vi "Is Possible.vi"(8 "error in (no error)":errorcluster, 10 "Cubes":T1, 11 "Bag in":refnum<class "Bag.lvclass">) -> (0 "error out":errorcluster, 2 "Compatible?":bool, 3 "Bag out":refnum<class "Bag.lvclass">)   [LabVIEW 2020, in "Bag.lvclass"]
uses:
  Bag.lvclass
  Cubes.ctl
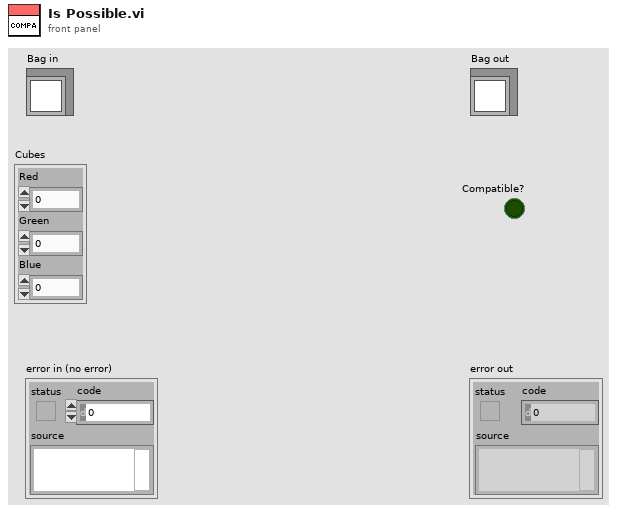
[diagram p1: front panel]
types:
  T1 = typedef "Bag.lvclass/Cubes.ctl" = cluster{"Red":i32, "Green":i32, "Blue":i32}
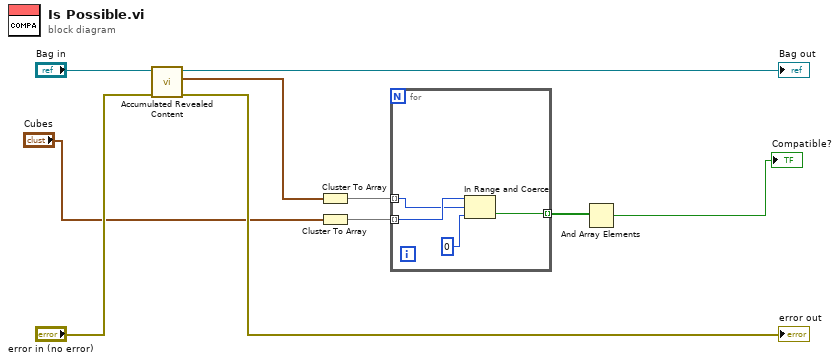
[diagram p0: block diagram]
diagram:
  n1 = call "Accumulated Revealed Content.vi"("error in (no error)"="error in (no error)", "Bag in"="Bag in") -> ("error out"=→"error out":errorcluster, "Cubes"=w6:T1, "Bag out"=→"Bag out":refnum<class "Bag.lvclass">)  [unwired: 7 in]
  n2 = Cluster To Array(cluster=w6) -> (array=w5:i32[])
  n3 = Cluster To Array(cluster="Cubes") -> (array=w3:i32[])
  n4 = for {
    tunnel: w5 -> [w11] mode=indexing
    tunnel: w3 -> [w12] mode=indexing
    tunnel: [w13] -> w2 mode=indexing
    n5 = In Range and Coerce(upper limit=w12, x=w11, lower limit=0) -> (In Range?=w13:bool)  [unwired: 1 out]
  }
  n6 = And Array Elements(Boolean array=w2) -> (logical AND=→"Compatible?":bool)
